vi "memory tree.vi"   [LabVIEW 2024, in "Nominal Client System Explorer.lvlib"]
uses:
  Nominal Client System Explorer.lvlib
  Built/Nominal Client/Windows/nominal-labview-client.lvlibp
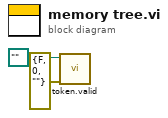
[diagram p0: block diagram]
diagram:
  n1 = call "token.valid.vi"("error in"=errorcluster {"status"=FALSE, "code"=0, "source"=""}, "token"=path "") -> ()  [unwired: 8 in, 2 out]
